vi "streamFromFile.vi"(8 "error in (no error)":errorcluster, 10 "Path":path, 11 "AnalogOutput in":refnum<class "AnalogOutput.lvclass">) -> (0 "error out":errorcluster, 3 "AnalogOutput out":refnum<class "AnalogOutput.lvclass">)   [LabVIEW 2009, in "Hardware.lvlib" / "Channels.lvlib" / "AnalogOutput.lvclass"]
uses:
  AnalogOutput.lvclass
  AnalogOutput.lvclass/AnalogOutput.ctl
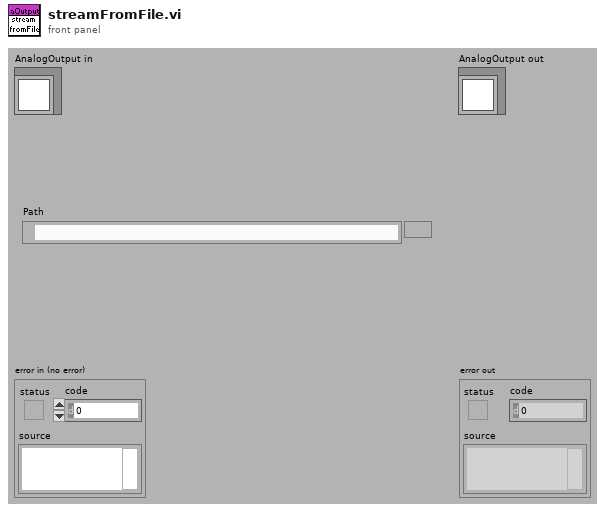
[diagram p1: front panel]
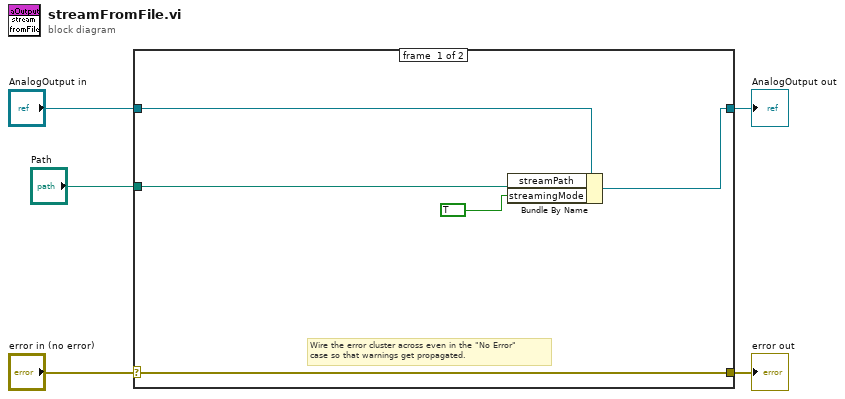
[diagram p0: block diagram]
diagram:
  n1 = case shown="No Error" "error in (no error)" {
    selector: "error in (no error)" -> [w10 w12]
    tunnel: [w10 w12] -> w4
    tunnel: [w8 w11] -> w2
    tunnel: "AnalogOutput in" -> [w9 w11]
    tunnel: "Path" -> [w7 _]
    frame #0 {
      # "Wire the error cluster across even in the \"No Error\"\ncase so that warnings get propagated."
      n2 = Bundle By Name(cluster=w9, "streamPath"=w7, "streamingMode"=TRUE) -> (w8:refnum<class "AnalogOutput.lvclass">)
    }
    frame #1 {
    }
  }
  "error out" <- w4
  "AnalogOutput out" <- w2
